vi "Create Execution Profiler Result View.vi"(8 "error in (no error)":errorcluster, 10 "Timing Results":map{string, dbl}(c390)) -> (0 "error out":errorcluster, 3 "Execution Profiler Result View out":refnum<class "Execution Profiler Result View.lvclass">)   [LabVIEW 2020, in "Execution Profiler.lvlib" / "Execution Profiler Result View.lvclass"]
uses:
  Execution Profiler Result View.lvclass
  Execution Profiler Result View.lvclass/Execution Profiler Result View.ctl
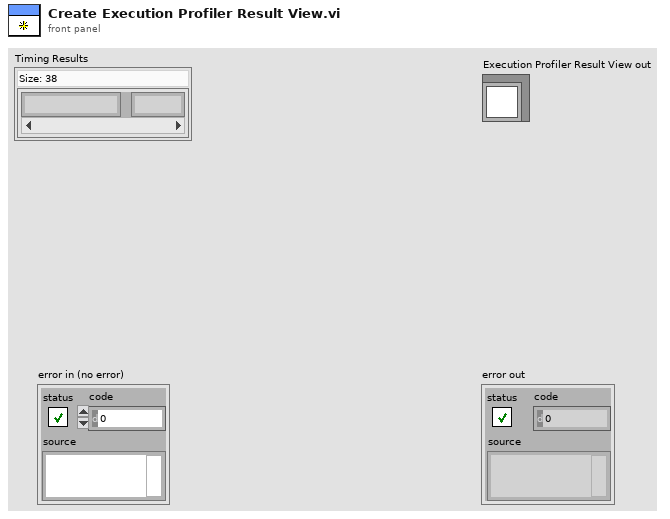
[diagram p1: front panel]
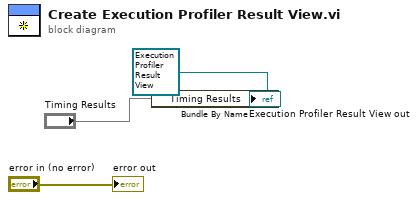
[diagram p0: block diagram]
diagram:
  n1 = Bundle By Name(cluster=refnum<class "Execution Profiler Result View.lvclass"> refnum ("Execution Profiler Result View out"), "Timing Results"="Timing Results") -> (→"Execution Profiler Result View out":refnum<class "Execution Profiler Result View.lvclass">)
  "error out" <- "error in (no error)"
